vi "Save Results.vi"(8 "error in (no error)":errorcluster, 10 "Results":refnum<class "Result.lvclass">[](array[class]), 11 "csv-formatter in":refnum<class "csv-formatter.lvclass">) -> (0 "error out":errorcluster, 3 "csv-formatter out":refnum<class "csv-formatter.lvclass">)   [LabVIEW 2015, in "csv-formatter.lvclass"]
doc: "This VI will take the array of results, format them and write them to the permanent report."
uses:
  csv-formatter.lvclass
  Result/Result.lvclass
  csv-formatter.lvclass/csv-formatter.ctl
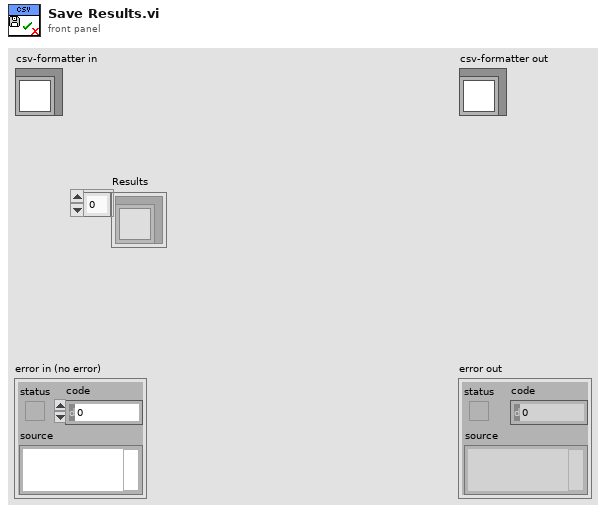
[diagram p1: front panel]
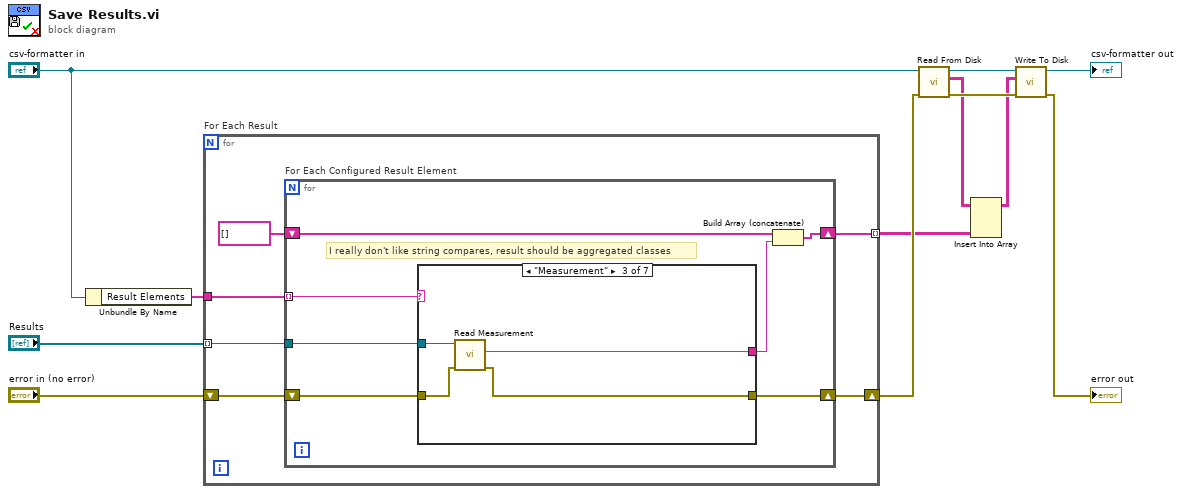
[diagram p0: block diagram]
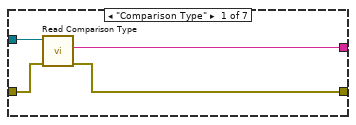
[diagram p2: hidden frame]
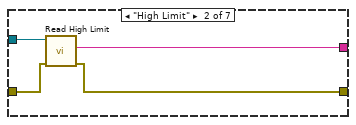
[diagram p3: hidden frame]
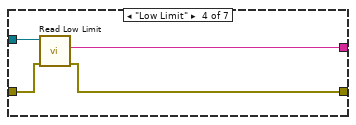
[diagram p4: hidden frame]
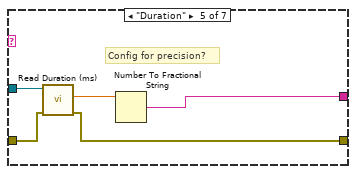
[diagram p5: hidden frame]
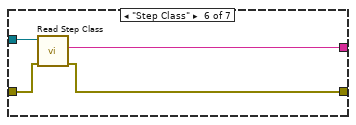
[diagram p6: hidden frame]
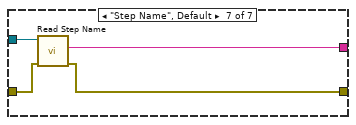
[diagram p7: hidden frame]
diagram:
  n1 = Unbundle By Name("csv-formatter in") -> ("Result Elements"=w10:string[])
  n2 = for "For Each Result" {
    tunnel: "Results" -> [w17] mode=indexing
    tunnel: w10 -> [w18]
    shift-right: [w15] -> w8
    shift-left: "error in (no error)" -> [w16]
    tunnel: [w13] -> w1 mode=indexing
    n3 = for "For Each Configured Result Element" {
      tunnel: w18 -> [w22] mode=indexing
      tunnel: w17 -> [w25]
      shift-right: [w23] -> w15
      shift-left: w16 -> [w24]
      shift-right: [w20] -> w13
      shift-left: string[] [] -> [w21]
      # "I really don't like string compares, result should be aggregated classes"
      n4 = case shown="\"Measurement\"" w22 {
        tunnel: w25 -> [w26 w33 w37 w41 w46 w50 w54]
        tunnel: w24 -> [w29 w32 w36 w40 w45 w49 w53]
        tunnel: [w28 w31 w35 w39 w44 w48 w52] -> w23
        tunnel: [w27 w30 w34 w38 w42 w47 w51] -> w19
        frame "Comparison Type" {
          n5 = call-dynamic "Read Comparison Type.vi"("error in (no error)"=w29, "Result in"=w26) -> ("error out"=w28:errorcluster, "Comparison Type"=w27:string)  [unwired: 7 in, 1 out]
        }
        frame "High Limit" {
          n6 = call-dynamic "Read High Limit.vi"("error in (no error)"=w32, "Result in"=w33) -> ("error out"=w31:errorcluster, "High Limit"=w30:string)  [unwired: 7 in, 1 out]
        }
        frame "Measurement" {
          n7 = call-dynamic "Read Measurement.vi"("error in (no error)"=w36, "Result in"=w37) -> ("error out"=w35:errorcluster, "Measurement"=w34:string)  [unwired: 7 in, 1 out]
        }
        frame "Low Limit" {
          n8 = call-dynamic "Read Low Limit.vi"("error in (no error)"=w40, "Result in"=w41) -> ("error out"=w39:errorcluster, "Low Limit"=w38:string)  [unwired: 7 in, 1 out]
        }
        frame "Duration" {
          # "Config for precision?"
          n9 = call-dynamic "Read Duration (ms).vi"("error in (no error)"=w45, "Result in"=w46) -> ("error out"=w44:errorcluster, "Duration (ms)"=w43:dbl)  [unwired: 7 in, 1 out]
          n10 = Number To Fractional String(number=w43) -> (F-format string=w42:string)  [unwired: 3 in]
        }
        frame "Step Class" {
          n11 = call-dynamic "Read Step Class.vi"("error in (no error)"=w49, "Result in"=w50) -> ("error out"=w48:errorcluster, "Step Class"=w47:string)  [unwired: 7 in, 1 out]
        }
        frame "Step Name", Default {
          n12 = call-dynamic "Read Step Name.vi"("error in (no error)"=w53, "Result in"=w54) -> ("error out"=w52:errorcluster, "Step Name"=w51:string)  [unwired: 7 in, 1 out]
        }
      }
      n13 = Build Array (concatenate)(w21, w19) -> (w20:string[])
    }
  }
  n14 = call "Read From Disk.vi"("error in (no error)"=w8, "csv-formatter in"="csv-formatter in") -> ("error out"=w6:errorcluster, "Result Out"=w3:string[][], "csv-formatter out"=w4:refnum<class "csv-formatter.lvclass">)  [unwired: 7 in]
  n15 = Insert Into Array(array=w3, new element=w1) -> (w2:string[][])  [unwired: 2 in]
  n16 = call "Write To Disk.vi"("error in (no error)"=w6, "Result In"=w2, "csv-formatter in"=w4) -> ("error out"=→"error out":errorcluster, "csv-formatter out"=→"csv-formatter out":refnum<class "csv-formatter.lvclass">)  [unwired: 7 in]
